vi "Initialize Routing Channel Page (State-Value Table).vi"(8 "error in (no error)":errorcluster, 10 "Routing Channel Page Controls":T1, 11 "Routing Channel Ref in":T2 format="%.0x") -> (0 "error out":errorcluster, 3 "Routing Channel Ref out":T2 format="%.0x")   [LabVIEW 2020, in "Routing and Faulting System Explorer.lvlib"]
uses:
  Routing and Faulting System Explorer.lvlib
  <vilib>/NI VeriStand/Custom Device API/Custom Device Item Ref.ctl
  Routing Channel Page Controls.ctl
  Routing Channel Initial Tab.ctl
  Scripting/Routing and Faulting Scripting.lvlib
  <vilib>/NI VeriStand/Custom Device API/Custom Device API.lvlib
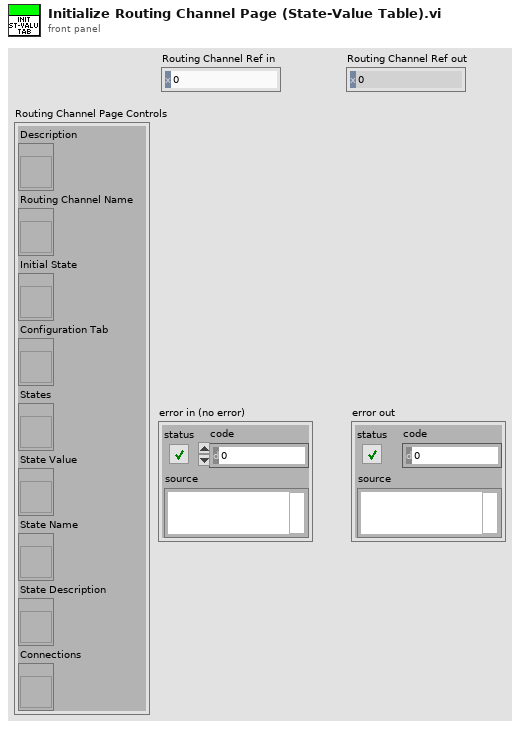
[diagram p1: front panel]
types:
  T1 = typedef "Routing and Faulting System Explorer.lvlib/Routing Channel Page Controls.ctl" = cluster{"Description":refnum<vi>, "Routing Channel Name":refnum<vi>, "Initial State":refnum<vi>, "Configuration Tab":refnum<vi>, "States":refnum<vi>, "State Value":refnum<vi>, "State Name":refnum<vi>, "State Description":refnum<vi>, "Connections":refnum<vi>}
  T2 = typedef "Custom Device API.lvlib/Custom Device Item Ref.ctl" = u64
  T3 = typedef "Routing and Faulting System Explorer.lvlib/Routing Channel Initial Tab.ctl" = enum16{"State Configuration", "State-Value Table", "State-Value Table if Empty"}
  T4 = enum8{"Enabled", "Disabled", "Disabled and Grayed Out"}
  T5 = enum32{"State Configuation", "State-Value Table"}
  T6 = enum32{"State Configuration", "State-Value Table"}
  T7 = typedef "Routing and Faulting System Explorer.lvlib/State-Value Row.ctl" = cluster{"State":string, "State Value":string}
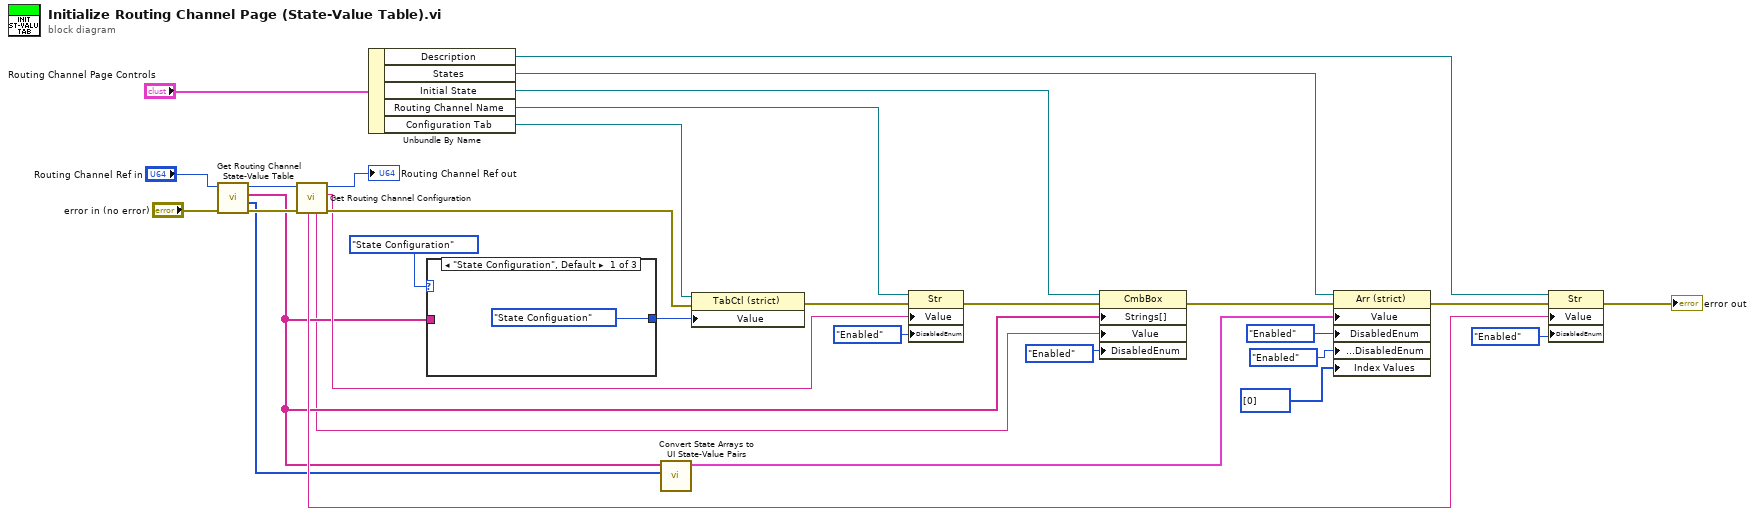
[diagram p0: block diagram]
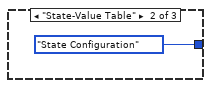
[diagram p2: hidden frame]
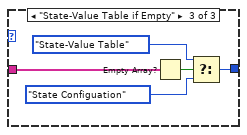
[diagram p3: hidden frame]
diagram:
  n1 = call "Get Routing Channel State-Value Table.vi"("error in"="error in (no error)", "routing channel in"="Routing Channel Ref in") -> ("error out"=w23:errorcluster, "state values"=w16:i32[], "state names"=w2:string[], "routing channel out"=w24:T2)  [unwired: 6 in]
  n2 = call "Get Routing Channel Configuration.vi"("error in"=w23, "routing channel in"=w24) -> ("error out"=w21:errorcluster, "routing channel name"=w20:string, "routing channel out"=→"Routing Channel Ref out":T2, "initial state"=w1:string, "description"=w29:string)  [unwired: 4 in, 1 out]
  n3 = Unbundle By Name("Routing Channel Page Controls") -> ("Description"=w28:refnum<vi>, "States"=w18:refnum<vi>, "Initial State"=w25:refnum<vi>, "Routing Channel Name"=w26:refnum<vi>, "Configuration Tab"=w27:refnum<vi>)
  n4 = case shown="\"State Configuration\", Default" Routing_Channel_Initial_Tab."State Configuration" ("Routing Channel Init Tab") {
    tunnel: [T5."State Configuation" ("Value") T6."State Configuration" ("Value") w37] -> w4
    tunnel: w2 -> [_ _ w36]
    frame "State Configuration", Default {
    }
    frame "State-Value Table" {
    }
    frame "State-Value Table if Empty" {
      n5 = Empty Array?(array=w36) -> (empty?=w38:bool)
      n6 = Select(t=T5."State-Value Table" ("Value"), s=w38, f=T5."State Configuation" ("Value")) -> (s? t:f=w37:T5)
    }
  }
  n7 = call "Convert State Arrays to UI State-Value Pairs.vi"("State Values"=w16, "State Names"=w2) -> ("State-Value Pairs"=w12:T7[])  [unwired: 9 in]
  n8 = property class="TabCtl (strict)"(reference=w27, error in=w21, "Value"=w4) -> (error out=w22:errorcluster)  [unwired: 1 out]
  n9 = property class="Str"(reference=w26, error in=w22, "Value"=w20, "DisabledEnum"=T4."Enabled" ("Array Element.Disabled")) -> (error out=w30:errorcluster)  [unwired: 1 out]
  n10 = property class="CmbBox"(reference=w25, error in=w30, "Strings[]"=w2, "Value"=w1, "DisabledEnum"=T4."Enabled" ("Array Element.Disabled")) -> (error out=w19:errorcluster)  [unwired: 1 out]
  n11 = property class="Arr (strict)"(reference=w18, error in=w19, "Value"=w12, "DisabledEnum"=T4."Enabled" ("Disabled"), "Array Element.DisabledEnum"=T4."Enabled" ("Array Element.Disabled"), "Index Values"=u32[] [0]) -> (error out=w17:errorcluster)  [unwired: 1 out]
  n12 = property class="Str"(reference=w28, error in=w17, "Value"=w29, "DisabledEnum"=T4."Enabled" ("Array Element.Disabled")) -> (error out=→"error out":errorcluster)  [unwired: 1 out]
